vi "GetOrCreateFlexChannel.vi"(8 "error in (no error)":errorcluster, 11 "Element Type":variant) -> (0 "error out":errorcluster, 2 "Channel Folder":path, 3 "Channel Control":path)   [LabVIEW 2020, in "FlexBlocks.lvlib"]
uses:
  FlexBlocks.lvlib
  <resource>/ChannelSupport/_ChannelScriptingSupport/_ChannelScriptingSupport.lvlib
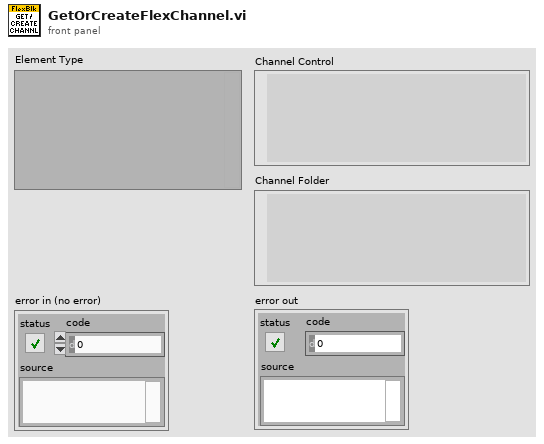
[diagram p1: front panel]
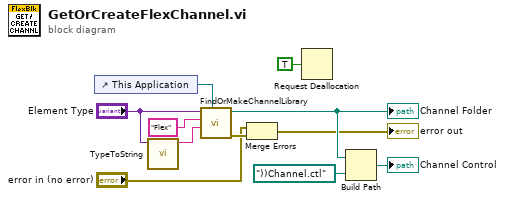
[diagram p0: block diagram]
diagram:
  n1 = control-ref of="This Application"() -> (w7:refnum<vi>)
  n2 = call <resource>:"TypeToString.vi"("type"="Element Type") -> ("string"=w10:string)  [unwired: 10 in]
  n3 = call <resource>:"FindOrMakeChannelLibrary.vi"("app"=w7, "typestring"=w10, "class"="Flex", "elt type"="Element Type") -> ("error out"=w3:errorcluster, "channel folder"=w9:path)  [unwired: 6 in]
  "Channel Folder" <- w9
  n4 = Merge Errors("error in (no error)", w3) -> (→"error out":errorcluster)
  n5 = Request Deallocation(TRUE ("flag")) -> ()
  n6 = Build Path(base path=w9, name or relative path=path "))Channel.ctl") -> (appended path=→"Channel Control":path)
